vi "Voltage Output Test.vi"(6 "Channel":i32=2, 7 "Signal Type":T1, 9 "Line in":dbl, 10 "Power Supply in":string, 11 "DMM in":string) -> (0 "error out":errorcluster, 3 "Output Voltage":dbl)   [LabVIEW 2025]
doc: "Measures the output DC voltage when providing an input voltage from the battery pins."
uses:
  Program Files (x86)/National Instruments/LabVIEW 2024/Instr.lib/Driver Simulation/DMM/Signal Types.ctl
  Program Files (x86)/National Instruments/LabVIEW 2024/Instr.lib/Driver Simulation/Power Supply.lvlib
  Program Files (x86)/National Instruments/LabVIEW 2024/Instr.lib/Driver Simulation/DMM.lvlib
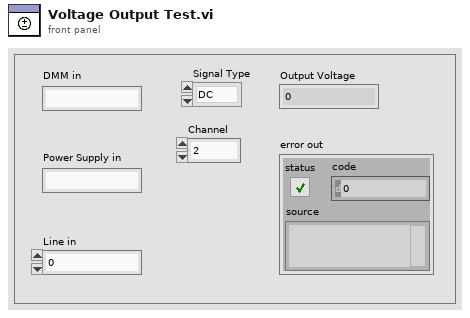
[diagram p1: front panel]
types:
  T1 = typedef "Driver Simulation.lvlib/DMM.lvlib/Signal Types.ctl" = enum16{"DC", "AC"}
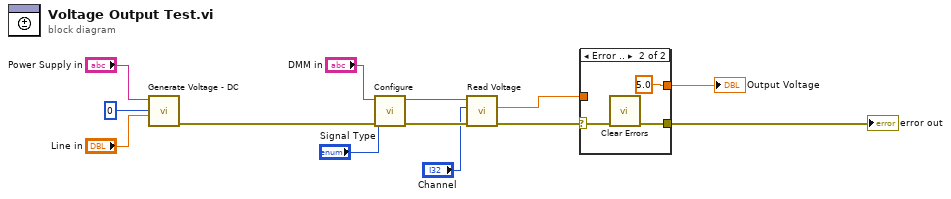
[diagram p0: block diagram]
diagram:
  n1 = call "Generate Voltage - DC.vi"("Output Voltage"="Line in", "Channel"=0, "Power Supply in"="Power Supply in") -> ("error out"=w13:errorcluster)  [unwired: 7 in, 1 out]
  n2 = call "Configure.vi"("error in (no error)"=w13, "Signal Type"="Signal Type", "DMM in"="DMM in") -> ("error out"=w12:errorcluster, "DMM out"=w5:string)  [unwired: 7 in]
  n3 = call "Read Voltage.vi"("error in (no error)"=w12, "Channel"="Channel", "DMM in"=w5) -> ("error out"=w4:errorcluster, "Voltage"=w3:dbl)  [unwired: 6 in, 1 out]
  n4 = case shown="Error .." w4 {
    selector: w4 -> [w14 w18]
    tunnel: w3 -> [w15 _]
    tunnel: [w15 5.0 ("Voltage")] -> w2
    tunnel: [w14 w16] -> w1
    frame No Error {
    }
    frame Error {
      n5 = call <vilib>:"Clear Errors.vi"("error in (no error)"=w18) -> ("error out"=w16:errorcluster)  [unwired: 5 in, 1 out]
    }
  }
  "error out" <- w1
  "Output Voltage" <- w2
